vi "File IO - FGV(V)_SubVIs-某型振动实验台测试系统.vi"(0 "Test Info":cluster{"Test Name":string, "Tester":string} caption="Test Information Input", 1 "Task Info.Accele Task":T1[](array[typedef]), 3 "Vibration Channel Name Input":string[](array[string]), 4 "文件路径":path, 5 "error in":errorcluster caption="Error In", 6 "Operation":T4, 7 "Chan":string="Vibration", 10 "测试条件":T2, 11 "粉尘特性":T3, 12 "Vibration Waveform":waveform(dbl)[](array[waveform])) -> (13 "粉尘特性 out":T3, 14 "Test Info":cluster{"Test Name":string, "Tester":string} caption="Test Information Output", 15 "Vibration Waveform":waveform(dbl)[](array[waveform]), 16 "units":string[](array[string]), 17 "测试条件out":T2, 18 "Vibration Chan Names Out":string[](array[string]), 19 "error out":errorcluster caption="Error out")   [LabVIEW 2011]
doc: "本VI是文件读写的功能性全局变量的范例，将对振动数据的TDMS文件的操作封装在一个子VI中。\n实现振动数据文件的创建、读取数据/实验信息、写入/实验信息、关闭等操作。"
panel:
  in  "Waveform Type":waveform(dbl)[](array[waveform])
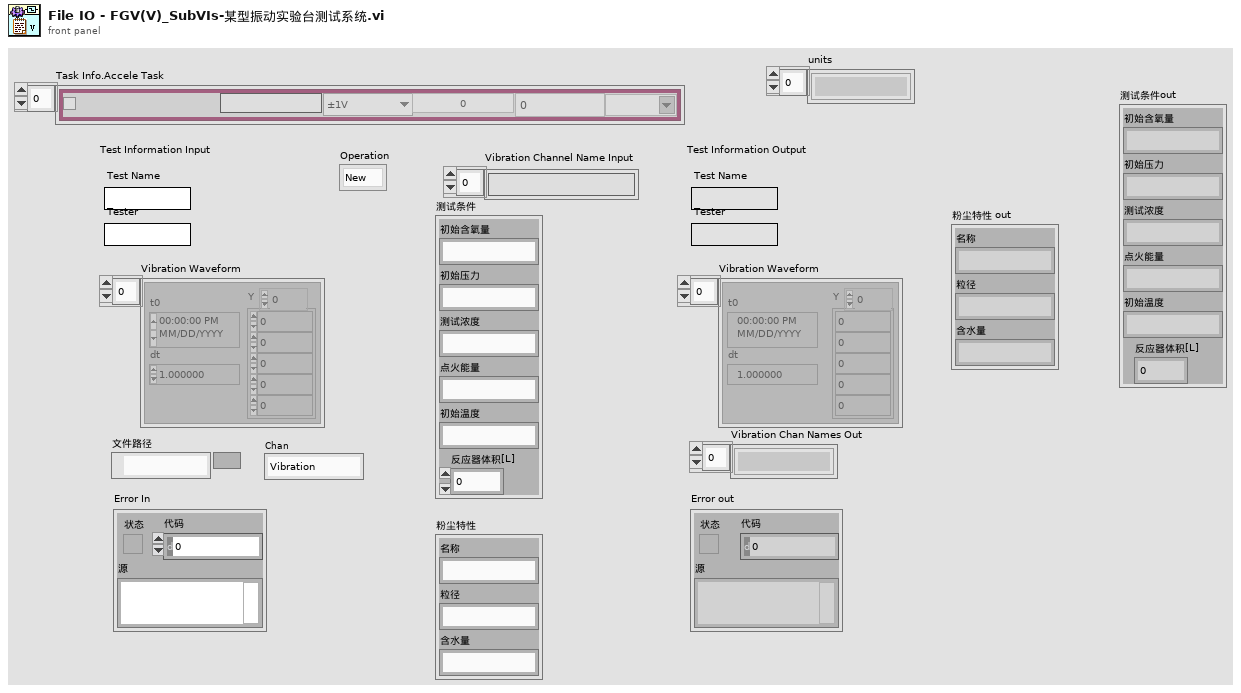
[diagram p1: front panel]
types:
  T1 = typedef "Acceleration Channel Config_Ctrls-某型振动实验台测试系统.ctl" = cluster{"Enable":bool, "Name":string, "range":enum16{"±1V", "±5V"}, "SensValue":dbl, "PhysicalName":string, "off":dbl, "Sensunits":string}
  T2 = typedef "测试条件.ctl" = cluster{"初始含氧量":string, "初始压力":string, "测试浓度":string, "点火能量":string, "初始温度":string, "反应器体积[L]":dbl}
  T3 = typedef "粉尘特性.ctl" = cluster{"名称":string, "粒径":string, "含水量":string}
  T4 = typedef "Enum File IO - FGV(V)_Ctrls-某型振动实验台测试系统.ctl" = enum16{"New", "Open", "Write Info", "Write Data", "Read Info", "Read Chan Names", "Read Data", "Close", "None"}
  T5 = enum16{"open", "open or create", "create or replace", "create", "open (read-only)"}
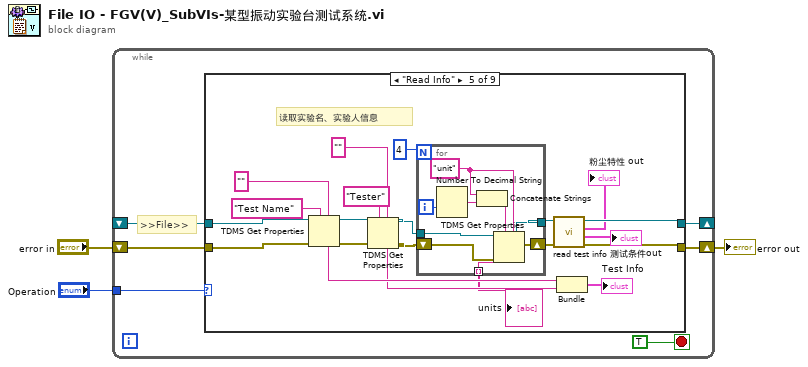
[diagram p0: block diagram]
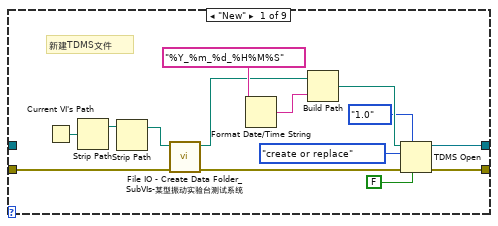
[diagram p2: hidden frame]
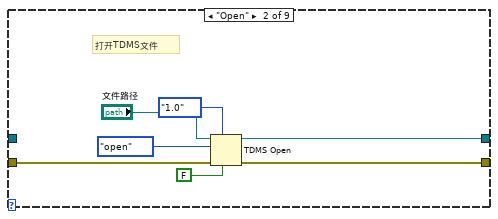
[diagram p3: hidden frame]
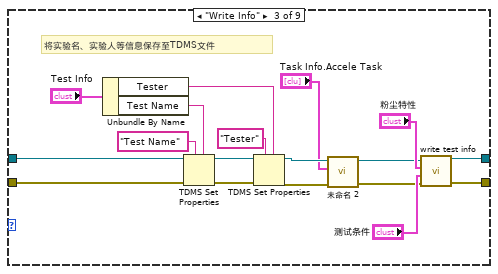
[diagram p4: hidden frame]
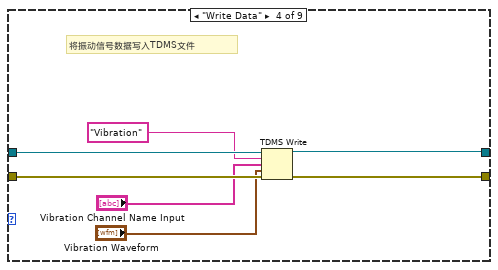
[diagram p5: hidden frame]
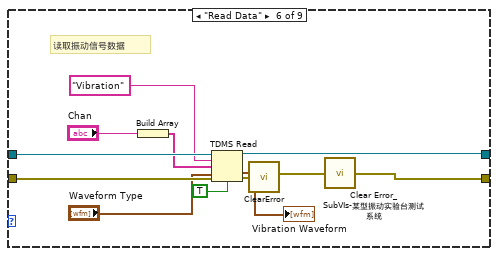
[diagram p6: hidden frame]
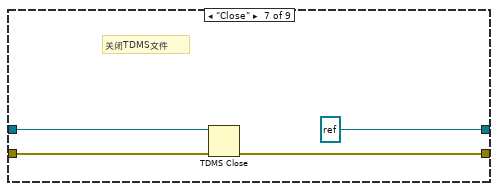
[diagram p7: hidden frame]
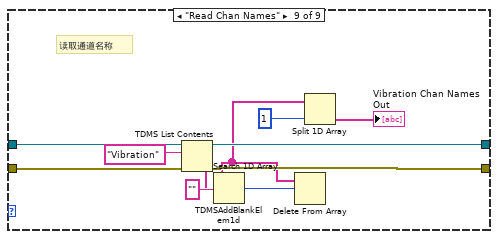
[diagram p9: hidden frame]
diagram:
  n1 = while {
    tunnel: "Operation" -> [w8]
    shift-right: [w6] -> w1
    shift-left: "error in" -> [w5]
    shift-right: [w7] -> _
    shift-left: _ -> [w4]
    stop <- TRUE stop-if-true
    # ">>File>>"
    n2 = case shown="\"Read Info\"" w8 {
      tunnel: [w23 w28 w39 w53 w64 w93 refnum<k34> refnum ("tdms file out") w103 w111] -> w7
      tunnel: [w20 w29 w38 w51 w65 w91 w98 w102 w112] -> w6
      tunnel: w5 -> [w16 w30 w48 w54 w76 w96 w101 w102 w113]
      tunnel: w4 -> [_ _ w47 w55 w68 w97 w100 w103 w114]
      frame "New" {
        # "新建TDMS文件"
        n3 = Current VI's Path() -> (path=w18:path)
        n4 = Strip Path(path=w18) -> (stripped path=w17:path)  [unwired: 1 out]
        n5 = Strip Path(path=w17) -> (stripped path=w15:path)  [unwired: 1 out]
        n6 = call "File IO - Create Data Folder_SubVIs-某型振动实验台测试系统.vi"("error in"=w16, "path input"=w15) -> ("error out"=w14:errorcluster, "path output"=w13:path)  [unwired: 8 out]
        n7 = Format Date/Time String(time format string (%c)="%Y_%m_%d_%H%M%S" ("时间格式字符串(%c)")) -> (date/time string=w12:string)  [unwired: 2 out]
        n8 = Build Path(base path=w13, name or relative path=w12) -> (appended path=w21:path)
        n9 = TDMS Open(6:FALSE ("禁用缓存(T)"), 7:enum16{"1.0", "2.0"}."1.0" ("文件格式版本(2.0)"), 8:w14, 10:T5."create or replace" ("操作(0:open)"), 11:w21) -> (0:w20:errorcluster, 3:w23:refnum<k34>)  [unwired: 1 in]
      }
      frame "Open" {
        # "打开TDMS文件"
        n10 = TDMS Open(6:FALSE ("禁用缓存(T)"), 7:enum16{"1.0", "2.0"}."1.0" ("文件格式版本(2.0)"), 8:w30, 10:T5."open" ("操作(0:open)"), 11:"文件路径") -> (0:w29:errorcluster, 3:w28:refnum<k34>)  [unwired: 1 in]
      }
      frame "Write Info" {
        # "将实验名、实验人等信息保存至TDMS文件"
        n11 = Unbundle By Name("Test Info") -> ("Tester"=w41:string, "Test Name"=w40:string)
        n12 = TDMS Set Properties(5:w40, 7:"Test Name", 8:w48, 11:w47) -> (0:w45:errorcluster, 3:w44:refnum<k34>)  [unwired: 4 out]
        n13 = TDMS Set Properties(5:w41, 7:"Tester", 8:w45, 11:w44) -> (0:w32:errorcluster, 3:w35:refnum<k34>)  [unwired: 4 out]
        n14 = call "未命名 2.vi"("错误输入（无错误）"=w32, "Task Info.Accele Task"="Task Info.Accele Task", "TDMS in"=w35) -> (0:w33:errorcluster, "TDMS out"=w34:refnum<k34>)  [unwired: 7 out]
        n15 = call "write test info.vi"("错误输入（无错误）"=w33, "测试条件"="测试条件", "粉尘特性"="粉尘特性", "tdms file in"=w34) -> ("错误输出"=w38:errorcluster, "TDMS文件输出"=w39:refnum<k34>)  [unwired: 6 out]
      }
      frame "Write Data" {
        # "将振动信号数据写入TDMS文件"
        n16 = TDMS Write(0:w55, 5:"Vibration" ("组名称输入（无标题）"), 7:"Vibration Channel Name Input", 9:"Vibration Waveform", 11:w54) -> (4:w53:refnum<k34>, 15:w51:errorcluster)  [unwired: 1 in, 2 out]
      }
      frame "Read Info" {
        # "读取实验名、实验人信息"
        n17 = TDMS Get Properties(5:"", 7:"Test Name", 8:w76, 11:w68) -> (0:w75:errorcluster, 3:w67:refnum<k34>, 4:w70:string)  [unwired: 5 out]
        n18 = TDMS Get Properties(5:"", 7:"Tester", 8:w75, 11:w67) -> (0:w61:errorcluster, 3:w58:refnum<k34>, 4:w66:string)  [unwired: 5 out]
        n19 = for {
          N: 4 -> [_]
          shift-right: [w79] -> w60
          shift-left: w61 -> [w78]
          tunnel: w58 -> [w84]
          tunnel: [w83] -> w57
          tunnel: [w80] -> w56 mode=indexing
          i -> [w85]
          w77 = "unit"
          n20 = Number To Decimal String(number=w85) -> (decimal integer string=w82:string)  [unwired: 1 out]
          n21 = Concatenate Strings(w77, w82) -> (w81:string)
          n22 = TDMS Get Properties(5:w77, 7:w81, 8:w78, 11:w84) -> (0:w79:errorcluster, 3:w83:refnum<k34>, 4:w80:string)  [unwired: 5 out]
        }
        "units" <- w56
        n23 = call "read test info.vi"("错误输入（无错误）"=w60, "tdms file in"=w57) -> ("错误输出"=w65:errorcluster, "测试条件"=→"测试条件out":T2, "粉尘特性"=→"粉尘特性 out":T3, "TDMS文件输出"=w64:refnum<k34>)  [unwired: 6 out]
        n24 = Bundle(w70, w66) -> (→"Test Info":cluster{string, string})  [unwired: 1 out]
      }
      frame "Read Data" {
        # "读取振动信号数据"
        n25 = Build Array("Chan") -> (w89:string[])
        n26 = TDMS Read(0:w97, 5:"Vibration" ("组名称输入（无标题）"), 7:w89, 11:w96, 12:"Waveform Type", 13:TRUE ("return channels in file order? (F)")) -> (4:w93:refnum<k34>, 10:→"Vibration Waveform":waveform(dbl)[], 15:w87:errorcluster)  [unwired: 2 in, 3 out]
        n27 = call <vilib>:"ClearError.vi"("error in (no error)"=w87) -> ("error out"=w88:errorcluster)
        n28 = call "Clear Error_SubVIs-某型振动实验台测试系统.vi"("error in (no error)"=w88) -> ("error out"=w91:errorcluster)
      }
      frame "Close" {
        # "关闭TDMS文件"
        n29 = TDMS Close(8:w101, 11:w100) -> (0:w98:errorcluster)  [unwired: 1 out]
      }
      frame "None", Default {
      }
      frame "Read Chan Names" {
        # "读取通道名称"
        n30 = TDMS List Contents(4:w113, 6:"Vibration" ("组名称输入（无标题）"), 7:w114) -> (0:w112:errorcluster, 1:w104:string[], 3:w111:refnum<k34>)  [unwired: 1 out]
        n31 = call <vilib>:"TDMSAddBlankElem1d.vi"("input string array"=w104) -> ("output string array with blank element at the beginning"=w105:string[])
        n32 = Search 1D Array(1D array=w105, element="") -> (index of element=w106:i32)  [unwired: 1 out]
        n33 = Delete From Array(array=w105, index=w106) -> ()  [unwired: 1 in, 2 out]
        n34 = Split 1D Array(array=w105, index=1) -> (second subarray=→"Vibration Chan Names Out":string[])  [unwired: 1 out]
      }
    }
  }
  "error out" <- w1
